vi "StepperControl.vi"() -> ()   [LabVIEW 2019]
uses:
  <vilib>/addons/control/pid/pid.llb/PID (DBL).vi
  <vilib>/addons/control/pid/NI_PID_pid.lvlib
  KNRm_ReMi_OS6_436Motor.lvlibp
panel:
  in  "PID gains":T1={"proportional gain (Kc)"=1.0, "integral time (Ti, min)"=0.01, "derivative time (Td, min)"=0.0} {"derivative time (Td, min)" format="%.3f"; "integral time (Ti, min)" format="%.3f"; "proportional gain (Kc)" format="%.3f"}
  in  "馬達現在位置":dbl
  in  "馬達未來目標":dbl
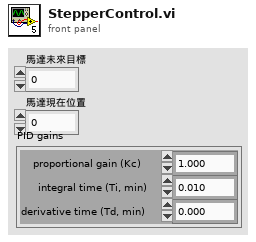
[diagram p1: front panel]
types:
  T1 = cluster{"proportional gain (Kc)":dbl, "integral time (Ti, min)":dbl, "derivative time (Td, min)":dbl}
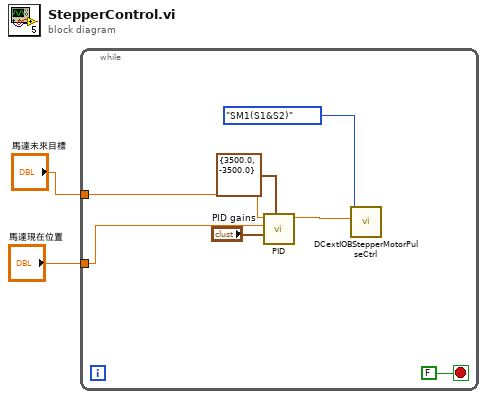
[diagram p0: block diagram]
diagram:
  n1 = while {
    tunnel: "馬達未來目標" -> [w8]
    tunnel: "馬達現在位置" -> [w9]
    stop <- FALSE stop-if-true
    n2 = call-poly <vilib>:"PID.vi"("output range"=cluster{"output high":dbl, "output low":dbl} {"output high"=3500.0, "output low"=-3500.0}, "PID gains"="PID gains", "process variable"=w9, "setpoint"=w8) -> ("output"=w4:dbl)  [unwired: 6 in, 1 out]
    n3 = call "DCextIOBStepperMotorPulseCtrl.vi"("PulseRate&Dir P/S"=w4, "Port"=enum16{"SM1(S1&S2)", "SM2(S3&S4)", "SM3(S5&S6)"}."SM1(S1&S2)") -> ()  [unwired: 8 in, 2 out]
  }
